vi "onAggregateResults.vi"(7 "Section":string, 8 "error in (no error)":errorcluster, 10 "Results":map{string, variant}(c390), 11 "Pips.TestResults in":refnum<class "Pips.TestResults.lvclass">) -> (0 "error out":errorcluster, 3 "Pips.TestResults out":refnum<class "Pips.TestResults.lvclass">)   [LabVIEW 2021, in "Banana.Caraya.lvlib" / "Pips.TestResults.lvclass"]
uses:
  Pips.TestResults.lvclass
  Pips.TestResults.lvclass/Pips.TestResults.ctl
  Bananas/Datastore.Dictionaries/Datastore.Dictionaries.lvclass
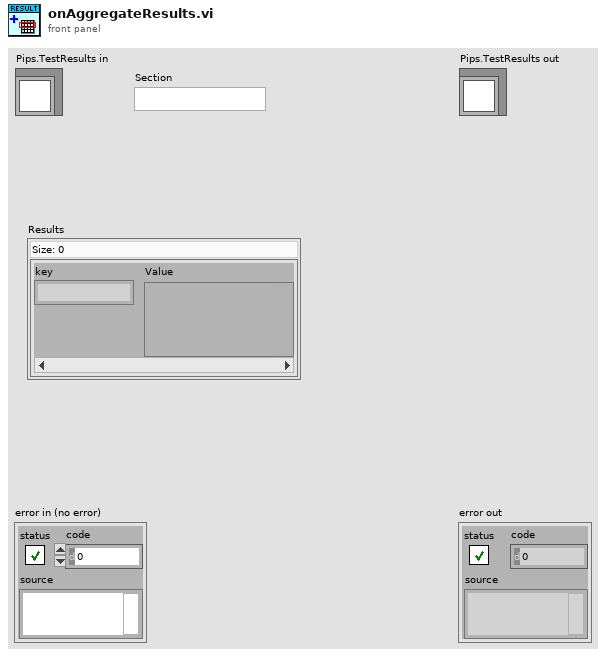
[diagram p1: front panel]
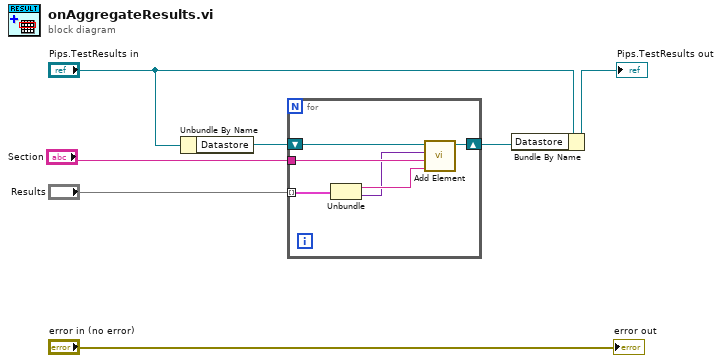
[diagram p0: block diagram]
diagram:
  n1 = Unbundle By Name("Pips.TestResults in") -> ("Datastore"=w4:refnum<class "Datastore.Dictionaries.lvclass">)
  n2 = for {
    shift-right: [w12] -> w3
    shift-left: w4 -> [w13]
    tunnel: "Section" -> [w11]
    tunnel: "Results" -> [w10] mode=indexing
    n3 = Unbundle(w10) -> ("key"=w9:string, "Value"=w8:variant)
    n4 = call "Add Element.vi"("element"=w9, "category"=w11, "Value"=w8, "Datastore.Dictionaries in"=w13) -> ("Datastore.Dictionaries"=w12:refnum<class "Datastore.Dictionaries.lvclass">)  [unwired: 5 in, 2 out]
  }
  n5 = Bundle By Name(cluster="Pips.TestResults in", "Datastore"=w3) -> (→"Pips.TestResults out":refnum<class "Pips.TestResults.lvclass">)
  "error out" <- "error in (no error)"
